vi "BATT-ABSOLUTE-Second.vi"(6 "B2":dbl, 7 "Comp":dbl, 9 "B1":dbl, 10 "A2":dbl, 11 "A1":dbl) -> (3 "Boolean":bool)   [LabVIEW 2016]
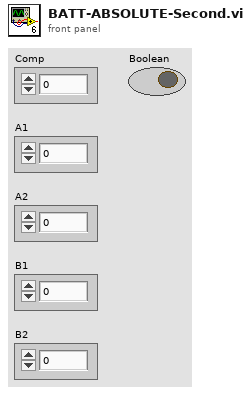
[diagram p1: front panel]
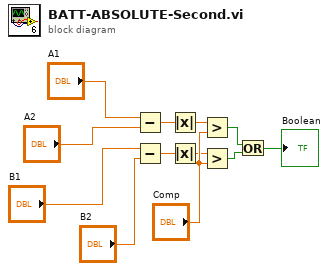
[diagram p0: block diagram]
diagram:
  n1 = Subtract(x="A1", y="A2") -> (x-y=w2:dbl)
  n2 = Subtract(x="B1", y="B2") -> (x-y=w4:dbl)
  n3 = Absolute Value(x=w2) -> (abs(x)=w1:dbl)
  n4 = Absolute Value(x=w4) -> (abs(x)=w3:dbl)
  n5 = Greater?(x=w1, y="Comp") -> (0:w6:bool)
  n6 = Greater?(x=w3, y="Comp") -> (0:w7:bool)
  n7 = Or(x=w6, y=w7) -> (x .or. y?=→"Boolean":bool)
